vi "CTRE_Phoenix_CANcoder_ConfigSensorInitializationStrategy.vi"(6 "timeoutMs":i32, 8 "error in":errorcluster, 10 "Sensor Initialization Strategy":T1, 11 "CTRE_CANcoder_DeviceRef":T2) -> (0 "error out":errorcluster, 3 "CTRE_CANcoder_DeviceRef":T2)   [LabVIEW 2020]
doc: "Sets the signage and range of the \"Absolute Position\" signal. \nChoose unsigned for an absolute range of [0,+1) rotations, [0,360) deg, etc...\nChoose signed for an absolute range of [-0.5,+0.5) rotations, [-180,+180) deg, etc...\n\n<b>Absolute Sensor Range </b> Desired Sign/Range for the absolute position register.\n<b>timeoutMs</b> Timeout value in ms. If nonzero, function will wait for config success and report an error if it times out. If zero, no blocking or checking is performed."
uses:
  <vilib>/Rock Robotics/WPI/ThirdParty/Phoenix-LabVIEW/CANCoder/Controls/CTRE_Phoenix_CANcoder_DeviceRef.ctl
  <vilib>/Rock Robotics/WPI/ThirdParty/Phoenix-LabVIEW/CANCoder/Controls/CTRE_Phoenix_CANcoder_SensorInitializationStrategy.ctl
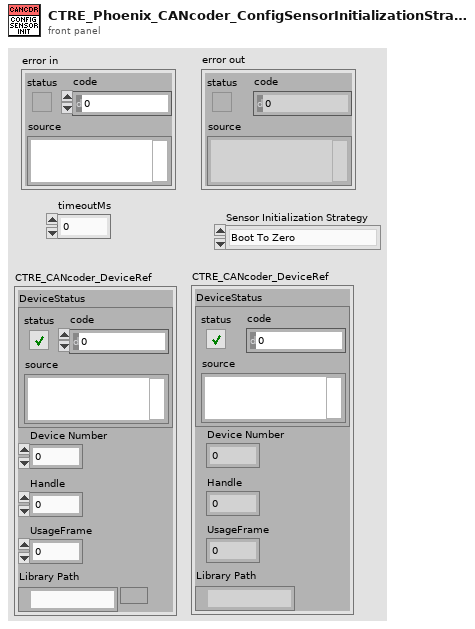
[diagram p1: front panel]
types:
  T1 = typedef "CTRE_Phoenix_CANcoder_SensorInitializationStrategy.ctl" = enum16{"Boot To Zero", "Boot To Absolute Position"}
  T2 = typedef "CTRE_Phoenix_CANcoder_DeviceRef.ctl" = cluster{"DeviceStatus":errorcluster, "Device Number":u8, "Handle":u64, "UsageFrame":u32, "Library Path":path}
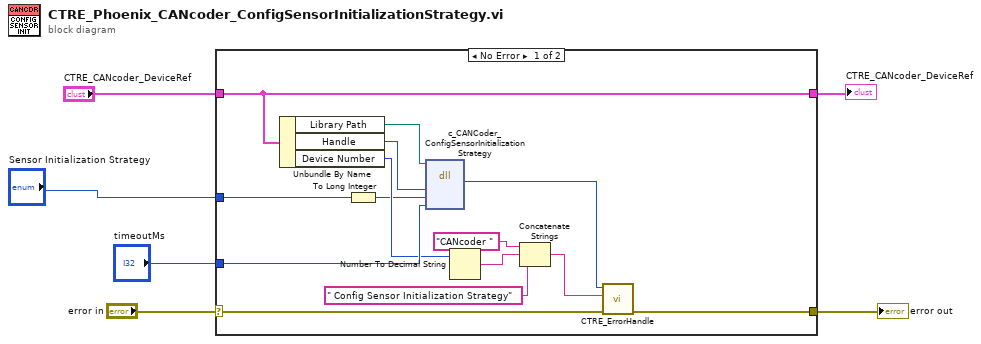
[diagram p0: block diagram]
diagram:
  n1 = case shown="No Error" "error in" {
    selector: "error in" -> [w17 w22]
    tunnel: "CTRE_CANcoder_DeviceRef" -> [w18 w21]
    tunnel: [w16 w22] -> w5
    tunnel: [w18 w21] -> w2
    tunnel: "timeoutMs" -> [w14 _]
    tunnel: "Sensor Initialization Strategy" -> [w7 _]
    frame No Error {
      n2 = Unbundle By Name(w18) -> ("Library Path"=w20:path, "Handle"=w19:u64, "Device Number"=w9:u8)
      n3 = To Long Integer(number=w7) -> (32bit integer=w8:i32)
      n4 = dll-call lib="?" fn="c_CANCoder_ConfigSensorInitializationStrategy"(path in=w20, "handle"=w19, "absoluteSensorRange"=w8, "timeoutMs"=w14) -> ("CTR_Code"=w15:i8)  [unwired: 5 in, 2 out]
      n5 = Number To Decimal String(number=w9) -> (decimal integer string=w13:string)  [unwired: 1 in]
      n6 = Concatenate Strings("CANcoder " ("string"), w13, " Config Sensor Initialization Strategy" ("string")) -> (w10:string)
      n7 = call <vilib>:"CTRE_ErrorHandle.vi"("error in"=w17, "origin"=w10, "code"=w15) -> ("error out"=w16:errorcluster)  [unwired: 8 in]
    }
    frame Error {
    }
  }
  "error out" <- w5
  "CTRE_CANcoder_DeviceRef" <- w2
